vi "_Dequeue JKISMQ.vi"(8 "Error in":errorcluster caption="Error in (no error)", 9 "Dequeue Timeout(0ms)":i32, 10 "State(s) in (\"\")":string, 11 "JKISMQ":T1) -> (0 "Error out":errorcluster, 2 "States Out":string, 3 "JKISMQ":T1)   [LabVIEW 2014, in "JKI-State-Machine-Plus.lvlib"]
uses:
  JKI-State-Machine-Plus.lvlib
  _JKISMQ.ctl
  _Cross JKI StateMachine State Data.ctl
  _Cross JKI StateMachine State Response.ctl
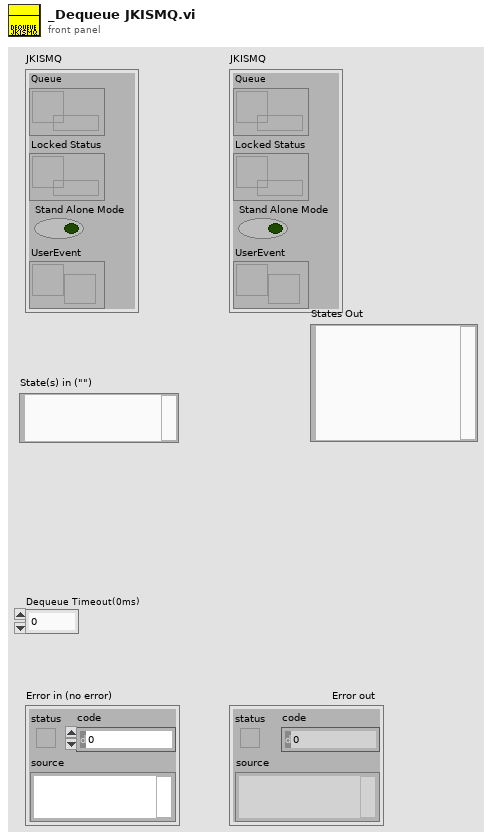
[diagram p1: front panel]
types:
  T1 = typedef "JKI-State-Machine-Plus.lvlib/_JKISMQ.ctl" = cluster{"Queue":refnum<queue>, "Locked Status":refnum<data-value>, "Stand Alone Mode":bool, "UserEvent":refnum<user-event>}
  T2 = typedef "JKI-State-Machine-Plus.lvlib/_Cross JKI StateMachine State Data.ctl" = cluster{"state":string, "args":string, "source":string, "RespQ":refnum<queue>}
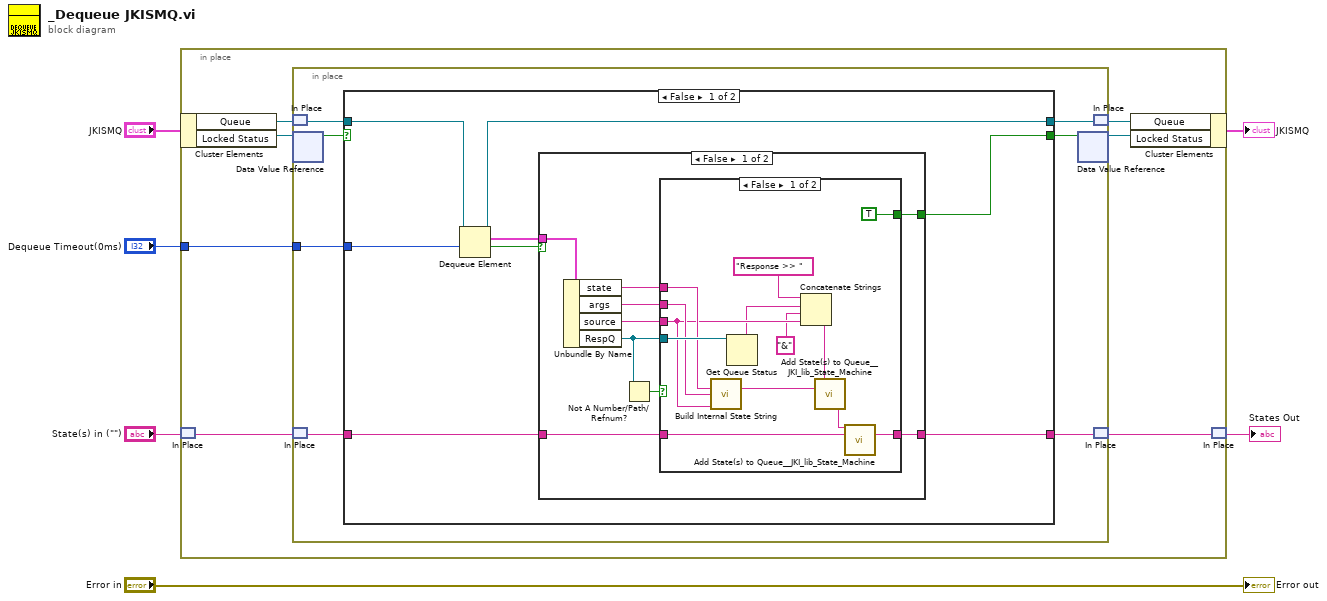
[diagram p0: block diagram]
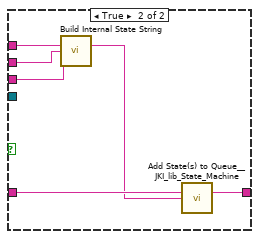
[diagram p2: hidden frame]
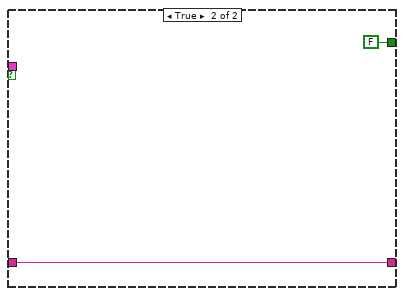
[diagram p3: hidden frame]
diagram:
  n1 = in-place "In Place Element Structure" {
    in-place-border: "Dequeue Timeout(0ms)" -> [w9]
    n2 = in-place-cluster #1("JKISMQ") -> ("Queue"=w13:refnum<queue>, "Locked Status"=w11:refnum<data-value>)
    n3 = in-place-match #2("State(s) in (\"\")") -> (w8:string)
    n4 = in-place {
      in-place-border: w9 -> [w18]
      n5 = in-place-match #3(w13) -> (w19:refnum<queue>)
      n6 = in-place-dvr #4(w11) -> (w17:bool)  [unwired: 1 out]
      n7 = in-place-match #5(w8) -> (w16:string)
      n8 = case shown="False" w17 {
        selector: w17 -> [_ w59]
        tunnel: [w27 w61] -> w20
        tunnel: w19 -> [w28 w61]
        tunnel: w18 -> [w26 _]
        tunnel: w16 -> [w23 w60]
        tunnel: [w22 w60] -> w15
        tunnel: [w21 w59] -> w14
        frame False {
          n9 = Dequeue Element(queue=w28, timeout in ms (-1)=w26) -> (queue out=w27:refnum<queue>, element=w24:T2, timed out?=w25:bool)  [unwired: 1 in, 1 out]
          n10 = case shown="False" w25 {
            tunnel: w23 -> [w36 w58]
            tunnel: [w35 w58] -> w22
            tunnel: w24 -> [w30 _]
            tunnel: [w29 FALSE] -> w21
            frame False {
              n11 = Unbundle By Name(w30) -> ("state"=w33:string, "args"=w32:string, "source"=w31:string, "RespQ"=w34:refnum<queue>)
              n12 = Not A Number/Path/Refnum?(number/path/refnum=w34) -> (NaN/Path/Refnum?=w37:bool)
              n13 = case shown="False" w37 {
                tunnel: w36 -> [w50 w56]
                tunnel: [w49 w55] -> w35
                tunnel: w34 -> [w48 _]
                tunnel: w33 -> [w43 w53]
                tunnel: w32 -> [w42 w52]
                tunnel: w31 -> [w41 w51]
                tunnel: [TRUE _] -> w29
                frame False {
                  n14 = call "Build Internal State String.vi"("State"=w43, "Arguments (\"\")"=w42, "Source (\"\")"=w41) -> ("State with Arguments"=w44:string)  [unwired: 12 in]
                  n15 = Get Queue Status(queue=w48) -> (queue name=w40:string)  [unwired: 2 in, 7 out]
                  n16 = Concatenate Strings("Response >> " ("State(s) at Back (\"\")"), w40, "&" ("string"), w41) -> (w45:string)
                  n17 = call <vilib>:"Add State(s) to Queue__JKI_lib_State_Machine.vi"("State(s) in (\"\")"=w44, "State(s) at Back (\"\")"=w45) -> ("States Out"=w47:string)  [unwired: 13 in]
                  n18 = call <vilib>:"Add State(s) to Queue__JKI_lib_State_Machine.vi"("State(s) in Front (\"\")"=w47, "State(s) in (\"\")"=w50) -> ("States Out"=w49:string)  [unwired: 13 in]
                }
                frame True {
                  n19 = call "Build Internal State String.vi"("State"=w53, "Arguments (\"\")"=w52, "Source (\"\")"=w51) -> ("State with Arguments"=w54:string)  [unwired: 12 in]
                  n20 = call <vilib>:"Add State(s) to Queue__JKI_lib_State_Machine.vi"("State(s) in (\"\")"=w56, "State(s) at Back (\"\")"=w54) -> ("States Out"=w55:string)  [unwired: 13 in]
                }
              }
            }
            frame True {
            }
          }
        }
        frame True {
        }
      }
      n21 = in-place-dvr #4(w14) -> (w10:refnum<data-value>)  [unwired: 1 out]
      n22 = in-place-match #3(w20) -> (w12:refnum<queue>)
      n23 = in-place-match #5(w15) -> (w7:string)
    }
    n24 = in-place-cluster #1("Queue"=w12, "Locked Status"=w10) -> (→"JKISMQ":T1)
    n25 = in-place-match #2(w7) -> (→"States Out":string)
  }
  "Error out" <- "Error in"
